vi "Draw.vi"(8 "error in (no error)":errorcluster, 10 "picture in (empty picture)":picture, 11 "Polygon in":refnum<class "Polygon.lvclass">) -> (0 "error out":errorcluster, 2 "picture out":picture, 3 "Polygon out":refnum<class "Polygon.lvclass">)   [LabVIEW 2018, in "Polygon.lvclass"]
doc: "Draw a rectangle"
uses:
  Polygon.lvclass
  Polygon.lvclass/Polygon.ctl
  Line/Line.lvclass
panel:
  # "expressionflow.com"
  # "Copyright (c) 2008 Tomi Maila. All rights reserved."
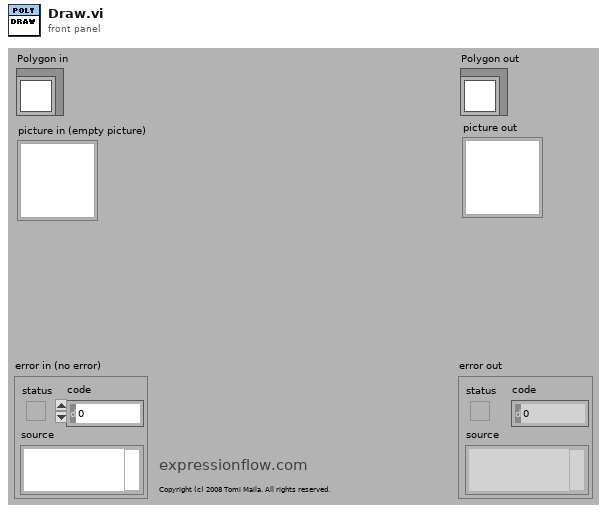
[diagram p1: front panel]
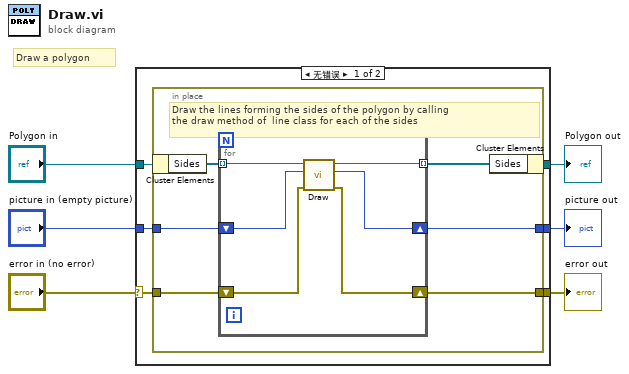
[diagram p0: block diagram]
diagram:
  # "Draw a polygon"
  n1 = case shown="无错误" "error in (no error)" {
    selector: "error in (no error)" -> [w11 w26]
    tunnel: [w8 w27] -> w5
    tunnel: "picture in (empty picture)" -> [w10 w27]
    tunnel: [w9 w26] -> w3
    tunnel: [w7 w25] -> w2
    tunnel: "Polygon in" -> [w12 w25]
    frame No Error {
      n2 = in-place {
        in-place-border: w11 -> [w14]
        in-place-border: w10 -> [w16]
        in-place-border: [w13] -> w9
        in-place-border: [w15] -> w8
        # "Draw the lines forming the sides of the polygon by calling \nthe draw method of  line class for each of the sides"
        n3 = in-place-cluster #1(w12) -> ("Sides"=w18:refnum<class "Line.lvclass">[])
        n4 = for {
          tunnel: w18 -> [w24] mode=indexing
          tunnel: [w23] -> w17 mode=indexing
          shift-right: [w21] -> w15
          shift-left: w16 -> [w22]
          shift-right: [w19] -> w13
          shift-left: w14 -> [w20]
          n5 = call-dynamic "Draw.vi"("error in (no error)"=w20, "picture in (empty picture)"=w22, "Line in"=w24) -> ("error out"=w19:errorcluster, "picture out"=w21:picture, "Line out"=w23:refnum<class "Line.lvclass">)  [unwired: 6 in]
        }
        n6 = in-place-cluster #1("Sides"=w17) -> (w7:refnum<class "Polygon.lvclass">)
      }
    }
    frame Error {
    }
  }
  "error out" <- w3
  "Polygon out" <- w2
  "picture out" <- w5
